vi "Time.FunctGlobal Timer.vi"(10 "Duration(s)":dbl, 11 "Action":T1) -> (0 "Remaining ms":i32, 1 "Done":bool, 2 "Progress(0-1)":dbl, 3 "Elapsed(s)":dbl, 4 "Remaining(s)":dbl)   [LabVIEW 2024, in "EQMF.lvlib" / "Time Utils.lvlib"]
doc: "This VI si a functional global timer.\nThe action input sets a duration and each time the Check action is used the status is outputted."
uses:
  Time Utils.lvlib
  Time.FunctGlobal Timer Action.ctl
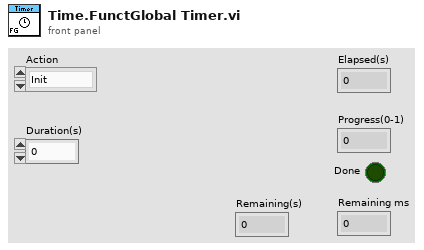
[diagram p1: front panel]
types:
  T1 = typedef "EQMF.lvlib/Time Utils.lvlib/Time.FunctGlobal Timer Action.ctl" = enum16{"Init", "Start", "Check", "Pause", "Resume", "Reset", "Stop"}
  T2 = cluster{"Running":bool, "Paused":bool, "Start":dbl, "Dur":dbl, "PausStart":dbl}
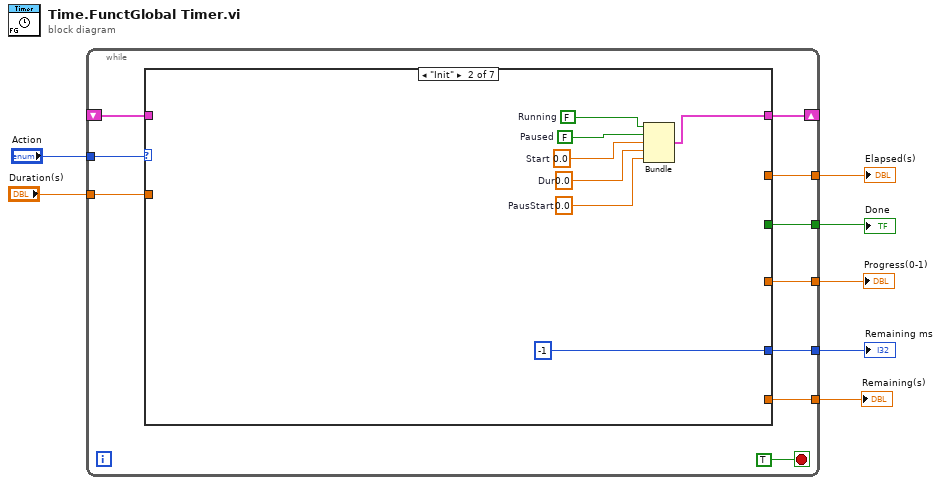
[diagram p0: block diagram]
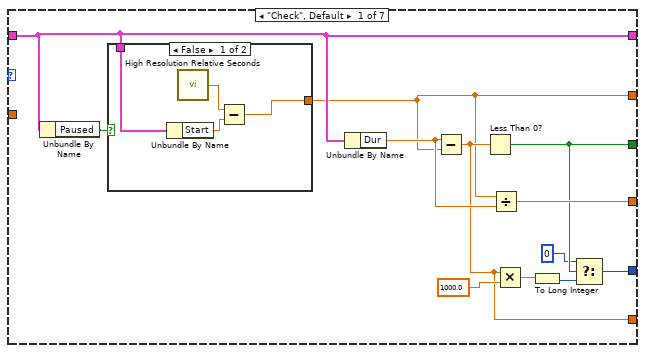
[diagram p2: hidden frame]
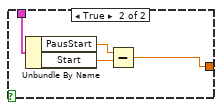
[diagram p3: hidden frame]
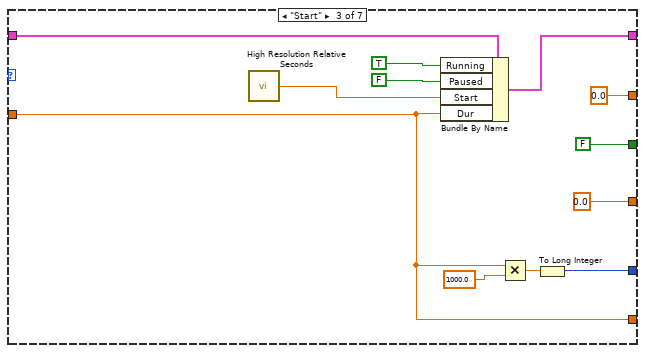
[diagram p4: hidden frame]
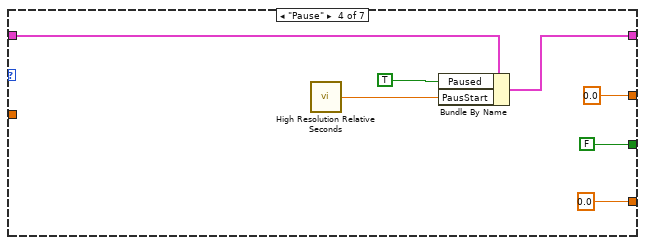
[diagram p5: hidden frame]
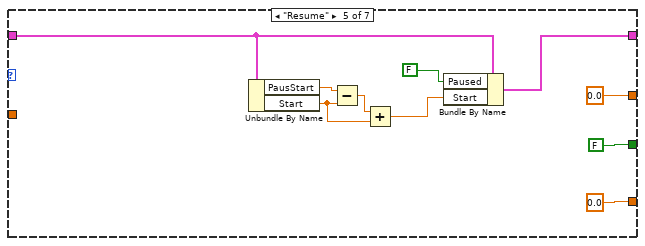
[diagram p6: hidden frame]
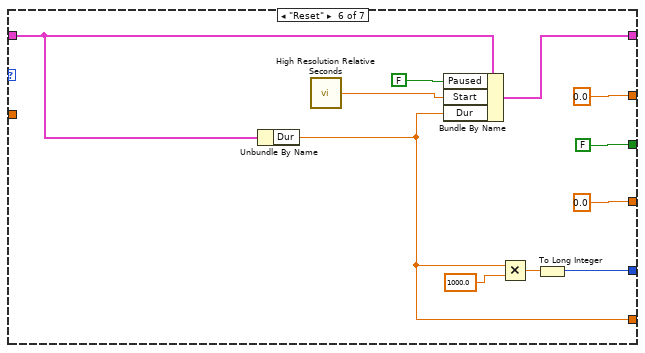
[diagram p7: hidden frame]
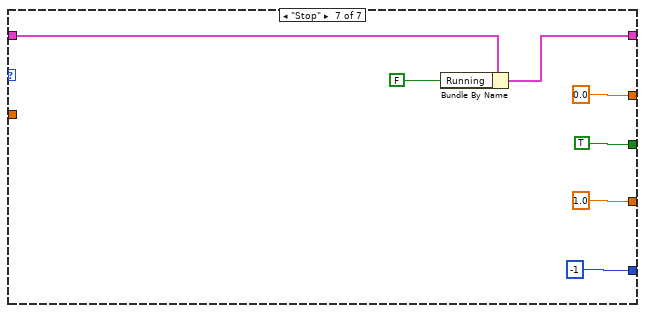
[diagram p8: hidden frame]
diagram:
  n1 = while {
    shift-right: [w16] -> _
    shift-left: _ -> [w14]
    tunnel: "Action" -> [w15]
    tunnel: [w13] -> w6
    tunnel: [w12] -> w5
    tunnel: [w11] -> w4
    tunnel: [w10] -> w3
    tunnel: "Duration(s)" -> [w9]
    tunnel: [w8] -> w1
    stop <- TRUE stop-if-true
    n2 = case shown="\"Init\"" w15 {
      tunnel: [w20 w40 w53 w61 w73 w82 w89] -> w16
      tunnel: w14 -> [w20 _ w56 w63 w68 w76 w91]
      tunnel: [w18 _ 0.0 0.0 0.0 0.0 0.0] -> w13
      tunnel: [w24 _ FALSE FALSE FALSE FALSE TRUE] -> w12
      tunnel: [w28 _ 0.0 0.0 0.0 0.0 1.0] -> w11
      tunnel: [w22 -1 w47 _ _ w77 -1] -> w10
      tunnel: w9 -> [_ _ w46 _ _ _ _]
      tunnel: [w21 _ w46 _ _ w74 _] -> w8
      frame "Check", Default {
        n3 = Unbundle By Name(w20) -> ("Paused"=w19:bool)
        n4 = case shown="False" w19 {
          tunnel: [w30 w34] -> w18
          tunnel: w20 -> [w33 w35]
          frame False {
            n5 = Unbundle By Name(w33) -> ("Start"=w31:dbl)
            n6 = call <vilib>:"High Resolution Relative Seconds.vi"() -> ("relative seconds"=w32:dbl)
            n7 = Subtract(x=w32, y=w31) -> (x-y=w30:dbl)
          }
          frame True {
            n8 = Unbundle By Name(w35) -> ("PausStart"=w37:dbl, "Start"=w36:dbl)
            n9 = Subtract(x=w37, y=w36) -> (x-y=w34:dbl)
          }
        }
        n10 = Unbundle By Name(w20) -> ("Dur"=w29:dbl)
        n11 = Subtract(x=w29, y=w18) -> (x-y=w21:dbl)
        n12 = Less Than 0?(x=w21) -> (x < 0?=w24:bool)
        n13 = Divide(x=w18, y=w29) -> (x/y=w28:dbl)
        n14 = Multiply(x=w21, y=1000.0) -> (x*y=w27:dbl)
        n15 = To Long Integer(number=w27) -> (32bit integer=w25:i32)
        n16 = Select(t=0, s=w24, f=w25) -> (s? t:f=w22:i32)
      }
      frame "Init" {
        w38 = FALSE  # Running
        w41 = 0.0  # PausStart
        w43 = 0.0  # Start
        w42 = 0.0  # Dur
        w44 = FALSE  # Paused
        n17 = Bundle("Running"=w38, "Paused"=w44, "Start"=w43, "Dur"=w42, "PausStart"=w41) -> (w40:T2)  [unwired: 1 in]
      }
      frame "Start" {
        n18 = call <vilib>:"High Resolution Relative Seconds.vi"() -> ("relative seconds"=w55:dbl)
        n19 = Bundle By Name(cluster=w56, "Running"=TRUE, "Paused"=FALSE ("Running"), "Start"=w55, "Dur"=w46) -> (w53:T2)
        n20 = Multiply(x=w46, y=1000.0) -> (x*y=w49:dbl)
        n21 = To Long Integer(number=w49) -> (32bit integer=w47:i32)
      }
      frame "Pause" {
        n22 = call <vilib>:"High Resolution Relative Seconds.vi"() -> ("relative seconds"=w62:dbl)
        n23 = Bundle By Name(cluster=w63, "Paused"=TRUE, "PausStart"=w62) -> (w61:T2)
      }
      frame "Resume" {
        n24 = Unbundle By Name(w68) -> ("PausStart"=w67:dbl, "Start"=w65:dbl)
        n25 = Subtract(x=w67, y=w65) -> (x-y=w66:dbl)
        n26 = Add(x=w66, y=w65) -> (x+y=w64:dbl)
        n27 = Bundle By Name(cluster=w68, "Paused"=FALSE, "Start"=w64) -> (w73:T2)
      }
      frame "Reset" {
        n28 = Unbundle By Name(w76) -> ("Dur"=w74:dbl)
        n29 = call <vilib>:"High Resolution Relative Seconds.vi"() -> ("relative seconds"=w84:dbl)
        n30 = Bundle By Name(cluster=w76, "Paused"=FALSE ("Running"), "Start"=w84, "Dur"=w74) -> (w82:T2)
        n31 = Multiply(x=w74, y=1000.0) -> (x*y=w75:dbl)
        n32 = To Long Integer(number=w75) -> (32bit integer=w77:i32)
      }
      frame "Stop" {
        n33 = Bundle By Name(cluster=w91, "Running"=FALSE) -> (w89:T2)
      }
    }
  }
  "Elapsed(s)" <- w6
  "Progress(0-1)" <- w4
  "Remaining ms" <- w3
  "Done" <- w5
  "Remaining(s)" <- w1
